vi "AppliedSettingsMatchStartPub.vi"(8 "error in (no error)":errorcluster, 10 "Applied?":bool, 11 "Model in":refnum<class "Model.lvclass">) -> (0 "error out":errorcluster, 3 "Model out":refnum<class "Model.lvclass">)   [LabVIEW 2016, in "Model.lvclass"]
uses:
  Model.lvclass
  Model.lvclass/Model.ctl
  PubSubDataEvent/PubSubDataEvent.lvclass/PubSubDataEvent.ctl
  PubSubDataEvent/PubSubDataEvent.lvclass
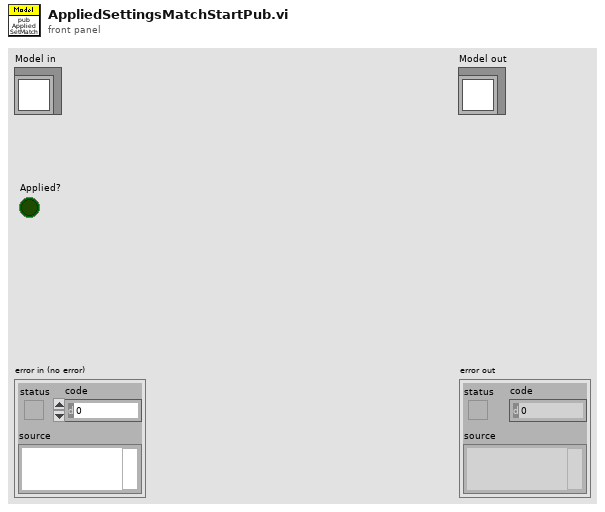
[diagram p1: front panel]
types:
  T1 = cluster{"appliedSettingsMatchStart":bool, "Timestamp":dbl}
  T2 = typedef "EXATypedefs.lvlib/PubDataEvents.ctl" = cluster{"AppliedSettingsMatchStart":refnum<user-event>, "SettingVersions":refnum<user-event>, "SummaryState":refnum<user-event>, "RejectedCommand":refnum<user-event>, "DetailedState":refnum<user-event>, "ErrorCode":refnum<user-event>, "Heartbeat":refnum<user-event>, "LoopTime_ms":refnum<user-event>, "LoopTimeOutOfRange":refnum<user-event>, "Timestamp":refnum<user-event>}
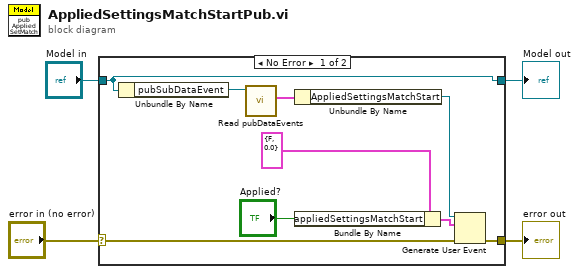
[diagram p0: block diagram]
diagram:
  n1 = case shown="No Error" "error in (no error)" {
    selector: "error in (no error)" -> [w6 w15]
    tunnel: "Model in" -> [w5 w14]
    tunnel: [w10 w15] -> w4
    tunnel: [w5 w14] -> w1
    frame No Error {
      n2 = Unbundle By Name(w5) -> ("pubSubDataEvent"=w13:refnum<class "PubSubDataEvent.lvclass">)
      n3 = call "Read pubDataEvents.vi"("PubSubDataEvent in"=w13) -> ("PubDataEvents"=w12:T2)  [unwired: 8 in, 2 out]
      n4 = Unbundle By Name(w12) -> ("AppliedSettingsMatchStart"=w11:refnum<user-event>)
      n5 = Bundle By Name(cluster=T1 {"appliedSettingsMatchStart"=FALSE, "Timestamp"=0.0} ("event data"), "appliedSettingsMatchStart"="Applied?") -> (w8:T1)
      n6 = Generate User Event(user event=w11, event data cluster=w8, error in=w6) -> (error out=w10:errorcluster)  [unwired: 1 in, 1 out]
    }
    frame Error {
    }
  }
  "error out" <- w4
  "Model out" <- w1
